vi "Get Visible State.vi"(8 "error in (no error)":errorcluster, 11 "JKI SM in":refnum<class "JKI SM.lvclass">) -> (0 "error out":errorcluster, 1 "State Name":string, 2 "Category":string, 3 "JKI SM out":refnum<class "JKI SM.lvclass">, 4 "is a Category Frame?":bool)   [LabVIEW 2013, in "JKI State Machine API.lvlib" / "JKI SM.lvclass"]
uses:
  JKI SM.lvclass
  JKI SM.lvclass/JKI SM.ctl
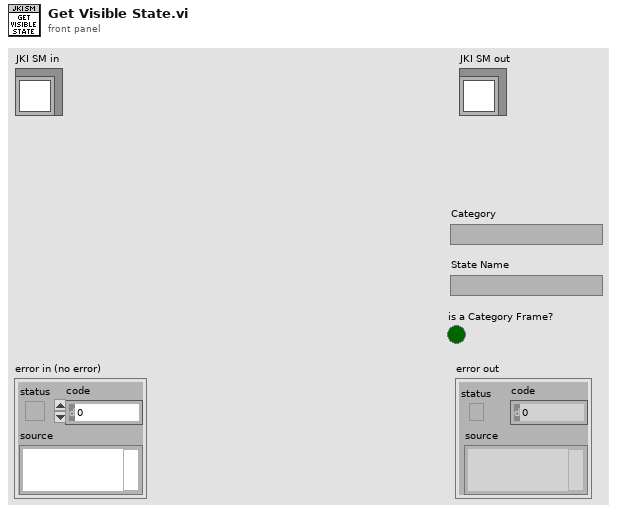
[diagram p1: front panel]
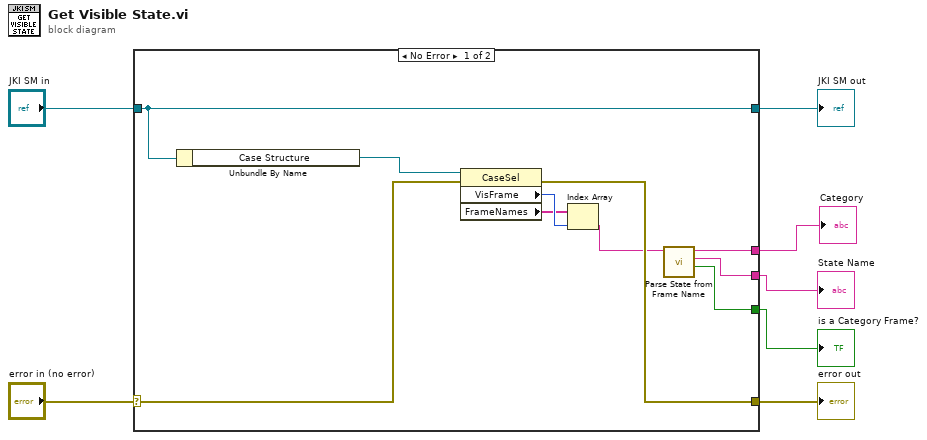
[diagram p0: block diagram]
diagram:
  n1 = case shown="No Error" "error in (no error)" {
    selector: "error in (no error)" -> [w14 w19]
    tunnel: [w17 w19] -> w6
    tunnel: [w15 w18] -> w4
    tunnel: "JKI SM in" -> [w15 w18]
    tunnel: [w10 _] -> w3
    tunnel: [w9 _] -> w2
    tunnel: [w8 _] -> w1
    frame No Error {
      n2 = Unbundle By Name(w15) -> ("Case Structure"=w16:refnum<vi>)
      n3 = property class="CaseSel"(reference=w16, error in=w14) -> (error out=w17:errorcluster, "VisFrame"=w13:u32, "FrameNames"=w12:string[])  [unwired: 1 out]
      n4 = Index Array(array=w12, index=w13) -> (element=w11:string)
      n5 = call "Parse State from Frame Name.vi"("Frame or State Name"=w11) -> ("is a Category Frame?"=w8:bool, "State Name"=w9:string, "Category Name"=w10:string)  [unwired: 6 in, 2 out]
    }
    frame Error {
    }
  }
  "error out" <- w6
  "JKI SM out" <- w4
  "State Name" <- w2
  "Category" <- w3
  "is a Category Frame?" <- w1
